vi "prepDOWaveplot.vi"(1 "DigitalGraph in":refnum<vi>, 2 "used DO names":string[](array[string])) -> ()   [LabVIEW 2015]
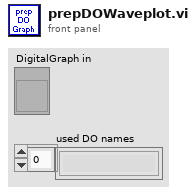
[diagram p1: front panel]
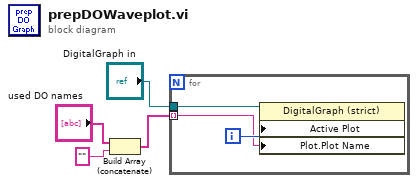
[diagram p0: block diagram]
diagram:
  n1 = Build Array (concatenate)("used DO names", "") -> (w1:string[])
  n2 = for {
    tunnel: w1 -> [w5] mode=indexing
    tunnel: "DigitalGraph in" -> [w6]
    i -> [w7]
    n3 = property on="Property Node" class="DigitalGraph (strict)"(reference=w6, "Active Plot"=w7, "Plot.Plot Name"=w5) -> ()  [unwired: 1 in, 2 out]
  }
